vi "Import PID Parameters.vi"(8 "error in":errorcluster) -> (0 "error out":errorcluster, 2 "Apply?":bool, 3 "Parameters":dbl[][](array[numeric]))   [LabVIEW 2013, in "Control Addon Shared.lvlib"]
uses:
  Control Addon Shared.lvlib
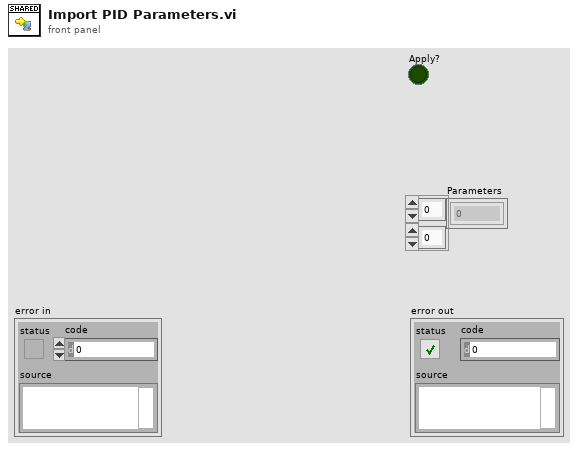
[diagram p1: front panel]
types:
  T1 = enum16{"open", "replace", "create", "open or create", "replace or create", "replace or create with confirmation"}
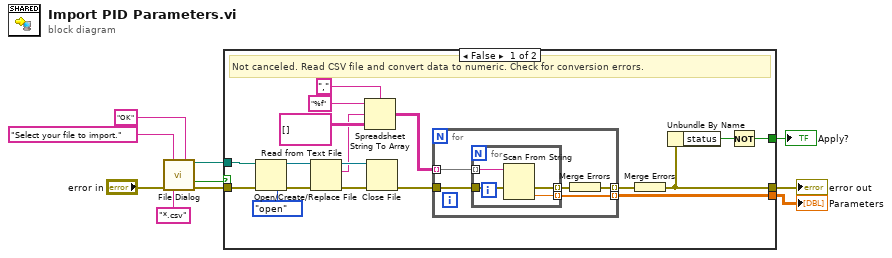
[diagram p0: block diagram]
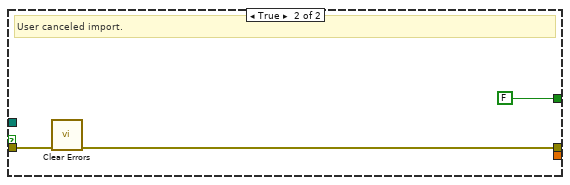
[diagram p2: hidden frame]
diagram:
  n1 = call "File Dialog"("prompt"="Select your file to import.", "button label"="OK", "error in"="error in", "pattern (all files)"="*.csv") -> ("selected path"=w6:path, "cancelled"=w9:bool, "error out"=w10:errorcluster)  [unwired: 8 in, 1 out]
  n2 = case shown="False" w9 {
    tunnel: w6 -> [w28 _]
    tunnel: w10 -> [w22 w40]
    tunnel: [w13 w38] -> w4
    tunnel: [w14 _] -> w2
    tunnel: [w11 FALSE] -> w1
    frame False {
      # "Not canceled. Read CSV file and convert data to numeric. Check for conversion errors."
      n3 = Open/Create/Replace File(file path (use dialog)=w28, error in=w22, operation (0:open)=T1."open") -> (refnum out=w27:refnum<file>, error out=w24:errorcluster)  [unwired: 3 in, 1 out]
      n4 = Read from Text File(file (use dialog)=w27, error in=w24) -> (refnum out=w25:refnum<file>, text=w16:string, error out=w26:errorcluster)  [unwired: 2 in, 1 out]
      n5 = Spreadsheet String To Array(delimiter (Tab)=",", format string="%f", spreadsheet string=w16, array type (2D Dbl)=string[][] []) -> (array=w20:string[][])
      n6 = Close File(refnum=w25, error in=w26) -> (error out=w17:errorcluster)  [unwired: 1 out]
      n7 = for {
        tunnel: w20 -> [w33] mode=indexing
        tunnel: [w32] -> w14 mode=indexing
        tunnel: [w31] -> w18 mode=indexing
        tunnel: w17 -> [w29]
        n8 = for {
          tunnel: w33 -> [w37] mode=indexing
          tunnel: [w36] -> w32 mode=indexing
          tunnel: [w35] -> w30 mode=indexing
          tunnel: w29 -> [w34]
          n9 = Scan From String(input string=w37, error in=w34) -> (error out=w35:errorcluster, output 1=w36:dbl)  [unwired: 3 in, 2 out]
        }
        n10 = Merge Errors(w30) -> (w31:errorcluster)
      }
      n11 = Merge Errors(w18) -> (w13:errorcluster)
      n12 = Unbundle By Name(w13) -> ("status"=w12:bool)
      n13 = Not(x=w12) -> (.not. x?=w11:bool)
    }
    frame True {
      # "User canceled import."
      n14 = call <vilib>:"Clear Errors.vi"("error in (no error)"=w40) -> ("error out"=w38:errorcluster)  [unwired: 6 in]
    }
  }
  "error out" <- w4
  "Parameters" <- w2
  "Apply?" <- w1
